vi "Remote Video snapshot.vi"(1 "Camera":T1="Travcam") -> (0 "Error out":errorcluster)   [LabVIEW 2015]
uses:
  Camera enum/Camera enum.ctl
  Globals/CamServer global.vi
panel:
  # "PN 27/08/15"
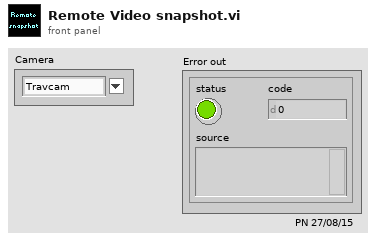
[diagram p1: front panel]
types:
  T1 = typedef "Camera enum.ctl" = string
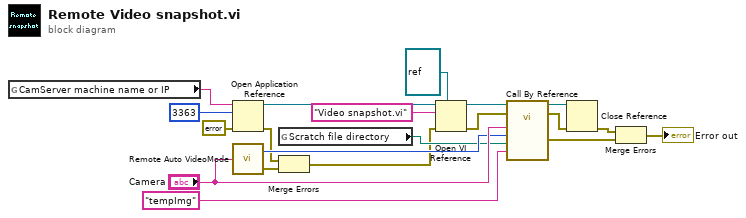
[diagram p0: block diagram]
diagram:
  n1 = global read "CamServer global.vi" "CamServer machine name or IP"() -> (w5:string)
  n2 = Open Application Reference(8:errorcluster {"status"=FALSE, "code"=0, "source"=""} ("error in (no error)"), 10:u16 3363 ("port"), 11:w5) -> (0:w3:errorcluster, 3:w18:refnum<vi>)  [unwired: 1 in]
  n3 = call "Remote Auto VideoMode.vi"("Camera"="Camera") -> ("VideoMode"=w8:u32, "Error out"=w2:errorcluster)
  n4 = global read "CamServer global.vi" "Scratch file directory"() -> (w4:path)
  n5 = Merge Errors(w3, w2) -> (w1:errorcluster)
  n6 = Open VI Reference(type specifier VI Refnum (for type only)=refnum<vi> refnum, application reference (local)=w18, vi path="Video snapshot.vi" ("machine name"), error in (no error)=w1) -> (vi reference=w16:refnum<vi>, error out=w17:errorcluster)  [unwired: 2 in]
  n7 = call-by-ref "?"(reference=w16, error in=w17, "Image name"="tempImg", "Image directory path"=w4, "VideoMode"=w8, "Interface name"="Camera") -> (reference out=w14:refnum<vi>, error out=w13:errorcluster, "Error Out"=w12:errorcluster)
  n8 = Close Reference(reference=w14, error in (no error)=w13) -> (error out=w11:errorcluster)
  n9 = Merge Errors(w11, w12) -> (→"Error out":errorcluster)
